vi "Find Tests.vi"(8 "error in (no error)":errorcluster, 10 "Project or Class Path":path, 11 "Execution UI In":refnum<class "Execution UI.lvclass">) -> (0 "error out":errorcluster, 3 "Execution UI Out":refnum<class "Execution UI.lvclass">)   [LabVIEW 2020, in "Execution UI.lvclass"]
uses:
  Execution UI.lvclass
  Execution UI.lvclass/Execution UI.ctl
  <vilib>/Comparison/Equal/Equal Functor/Equal Functor.lvclass
  Framework/Test Finder/Test Finder.lvclass
  Result Model by Reference/Result Model by Reference.lvclass
  LUnit Test Suite.lvclass
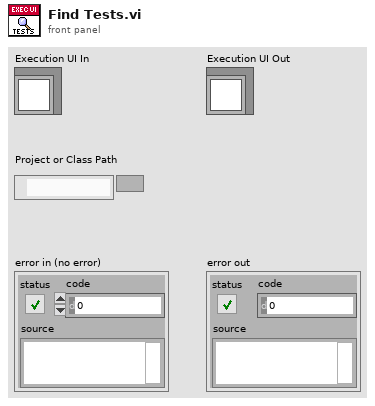
[diagram p1: front panel]
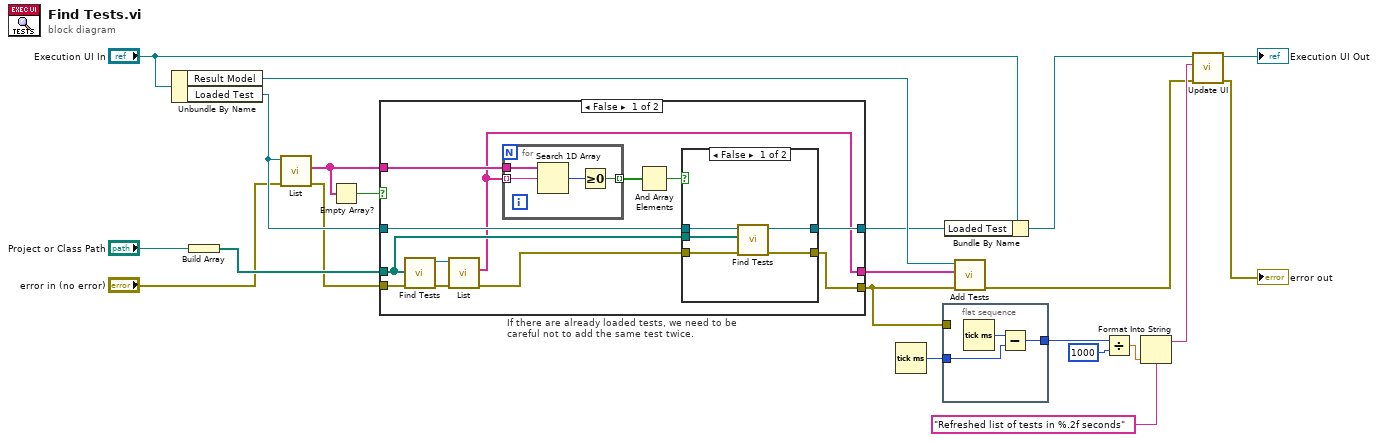
[diagram p0: block diagram]
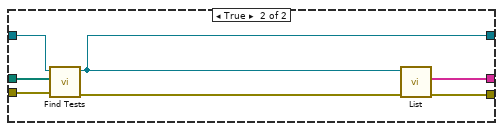
[diagram p3: hidden frame]
diagram:
  n1 = Unbundle By Name("Execution UI In") -> ("Result Model"=w9:refnum<class "Result Model by Reference.lvclass">, "Loaded Test"=w6:refnum<class "LUnit Test Suite.lvclass">)
  n2 = Build Array("Project or Class Path") -> (w14:path[])
  n3 = call "List.vi"("error in (no error)"="error in (no error)", "LUnit Test Suite In"=w6) -> ("error out"=w4:errorcluster, "List of Runnables"=w2:string[])  [unwired: 8 in]
  n4 = Empty Array?(array=w2) -> (empty?=w3:bool)
  n5 = case "If there are already loaded tests, we need to be careful not to add the same test twice." shown="False" w3 {
    tunnel: [w25 w48] -> w16
    tunnel: w14 -> [w24 w52]
    tunnel: [w29 w47] -> w7
    tunnel: w6 -> [w28 w51]
    tunnel: w4 -> [w33 w50]
    tunnel: w2 -> [w34 _]
    tunnel: [w23 w46] -> w1
    frame False {
      n6 = call "Find Tests.vi"("error in (no error)"=w33, "File Paths"=w24) -> ("error out"=w31:errorcluster, "LUnit Test Suite"=w32:refnum<class "LUnit Test Suite.lvclass">)  [unwired: 8 in]
      n7 = call "List.vi"("error in (no error)"=w31, "LUnit Test Suite In"=w32) -> ("error out"=w26:errorcluster, "List of Runnables"=w23:string[])  [unwired: 8 in]
      n8 = for {
        tunnel: w34 -> [w38]
        tunnel: w23 -> [w37] mode=indexing
        tunnel: [w35] -> w30 mode=indexing
        n9 = Search 1D Array(1D array=w38, element=w37) -> (index of element=w36:i32)  [unwired: 1 in]
        n10 = Greater Or Equal To 0?(x=w36) -> (x >= 0?=w35:bool)
      }
      n11 = And Array Elements(Boolean array=w30) -> (logical AND=w27:bool)
      n12 = case shown="False" w27 {
        tunnel: [w43 w45] -> w29
        tunnel: w28 -> [w42 w45]
        tunnel: w26 -> [w41 w44]
        tunnel: [w40 w44] -> w25
        tunnel: w24 -> [w39 _]
        frame False {
          n13 = call "Find Tests.vi"("error in (no error)"=w41, "File Paths"=w39, "LUnit Test Suite"=w42) -> ("error out"=w40:errorcluster, "LUnit Test Suite"=w43:refnum<class "LUnit Test Suite.lvclass">)  [unwired: 7 in]
        }
        frame True {
        }
      }
    }
    frame True {
      n14 = call "Find Tests.vi"("error in (no error)"=w50, "File Paths"=w52, "LUnit Test Suite"=w51) -> ("error out"=w49:errorcluster, "LUnit Test Suite"=w47:refnum<class "LUnit Test Suite.lvclass">)  [unwired: 7 in]
      n15 = call "List.vi"("error in (no error)"=w49, "LUnit Test Suite In"=w47) -> ("error out"=w48:errorcluster, "List of Runnables"=w46:string[])  [unwired: 8 in]
    }
  }
  n16 = Tick Count (ms)() -> (millisecond timer value=w22:u32)
  n17 = flat-sequence {
    tunnel: w22 -> [w55]
    tunnel: [w54] -> w20
    tunnel: w16 -> [_]
    frame #0 {
      n18 = Tick Count (ms)() -> (millisecond timer value=w53:u32)
      n19 = Subtract(x=w53, y=w55) -> (x-y=w54:u32)
    }
  }
  n20 = Bundle By Name(cluster="Execution UI In", "Loaded Test"=w7) -> (w13:refnum<class "Execution UI.lvclass">)
  n21 = call "Add Tests.vi"("error in (no error)"=w16, "Tests"=w1, "Result Model by Reference In"=w9) -> ("error out"=w8:errorcluster)  [unwired: 8 in]
  n22 = Divide(x=w20, y=u32 1000) -> (x/y=w21:dbl)
  n23 = Format Into String(format string="Refreshed list of tests in %.2f seconds" ("Status"), w21) -> (resulting string=w17:string)  [unwired: 2 in, 1 out]
  n24 = call "Update UI.vi"("error in (no error)"=w8, "Status"=w17, "Execution UI In"=w13) -> ("error out"=→"error out":errorcluster, "Execution UI Out"=→"Execution UI Out":refnum<class "Execution UI.lvclass">)  [unwired: 7 in]
